vi "Test-Multiplier Glide.vi"() -> ()   [LabVIEW 2020, in "Level.lvclass"]
uses:
  Level.lvclass
panel:
  out "Waveform Graph":dbl[](graph)
  in  "new mult":dbl format="%#_13g"
  in  "last mult":dbl format="%#_13g"
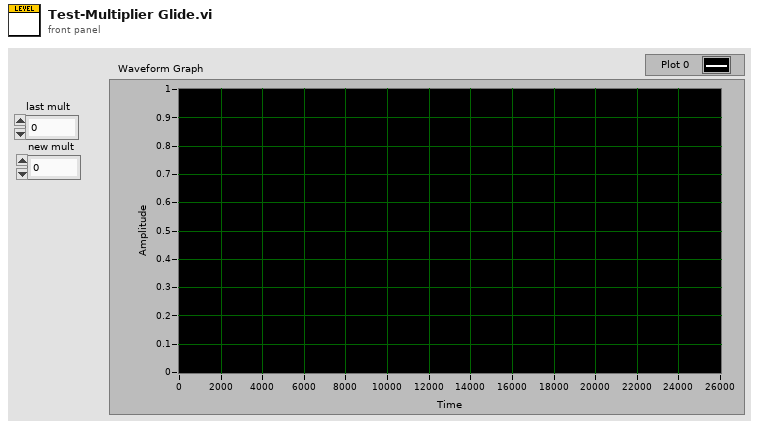
[diagram p1: front panel]
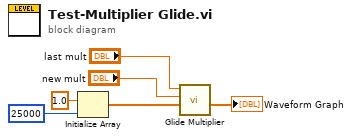
[diagram p0: block diagram]
diagram:
  n1 = Initialize Array(1.0 ("element"), 25000 ("dimension size")) -> (w4:dbl[])
  n2 = call "Glide Multiplier.vi"("Array in"=w4, "new mult"="new mult", "last mult"="last mult") -> ("Array out"=→"Waveform Graph":dbl[])  [unwired: 4 in]
